vi "write_rois_to_results_file.vi"(8 "Error In":errorcluster, 9 "ROIs":T1(array[cluster]), 10 "Sample":string, 11 "File Path":path) -> (0 "Error Out":errorcluster)   [LabVIEW 2019]
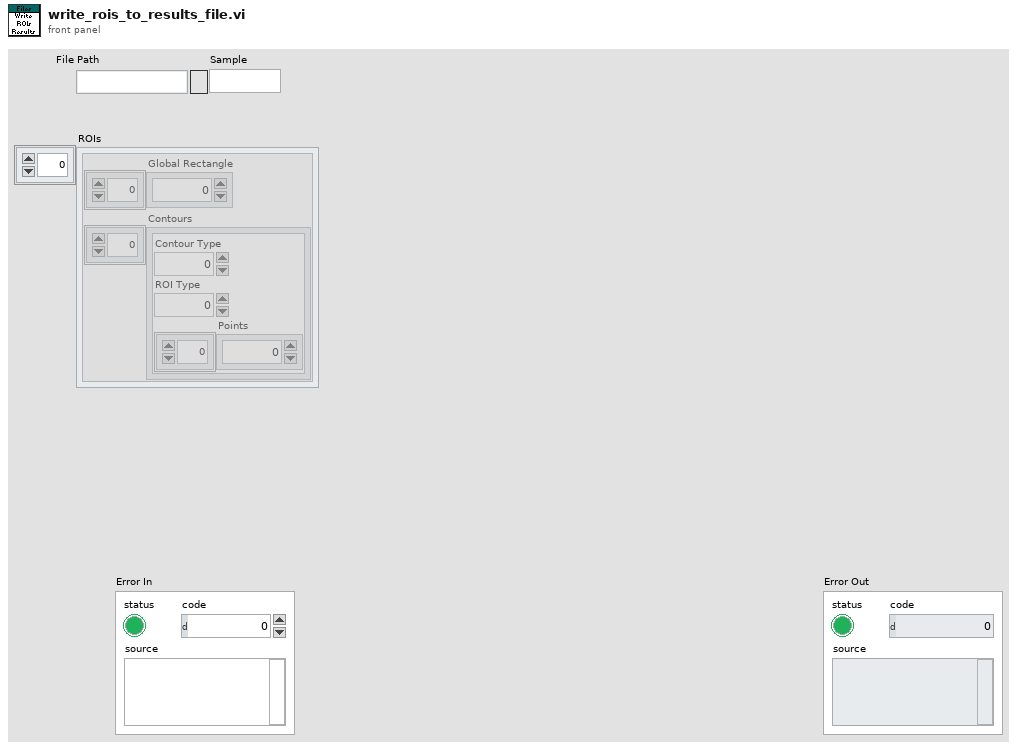
[diagram p1: front panel]
types:
  T1 = cluster{"Global Rectangle":i32[], "Contours":cluster{"Contour Type":u32, "ROI Type":u32, "Points":i32[]}[]}[]
  T2 = typedef "sample_results_cluster_typedef.ctl" = cluster{"File Path":string, "Sample":string, "Threshold":dbl, "Parameters":T3, "Writeable Parameters":T4, "Gain Results":T5[]}
  T3 = typedef "parameters_cluster_typedef.ctl" = cluster{"m1":dbl, "m2":dbl, "m3":dbl, "c":dbl, "D":dbl, "Beta":dbl, "center x":dbl, "center y":dbl}
  T4 = typedef "writeable_section_parameters_cluster_typedef.ctl" = cluster{"Section":string, "Method":i32, "Edge Mode":i32, "Grid Constant":i32, "Manual Sequence":i32, "ROI Size":i32, "Min Grain Size":dbl, "Comments":string, "File Path":string}
  T5 = typedef "grain_results_cluster_typedef.ctl" = cluster{"Grain Number":i32, "xi":dbl[], "phiin":dbl[], "Intensity":dbl[][], "Best Fit Intensity":dbl[][], "Best Fit Parameters":dbl[][], "Polarizer 1 Angle":dbl[][], "Polarizer 2 Angle":dbl[][], "Best Extinction Angle":dbl[], "Best Extinction Angle Corrected":dbl[], "Thetac":dbl, "Phic":dbl, "ROI":cluster{"Global Rectangle":i32[], "Contours":cluster{"Contour Type":u32, "ROI Type":u32, "Points":i32[]}[]}, "a":dbl, "b":dbl, "sequences available":dbl, "sequences used":dbl, "Contrast":dbl[], "Rsq":dbl}
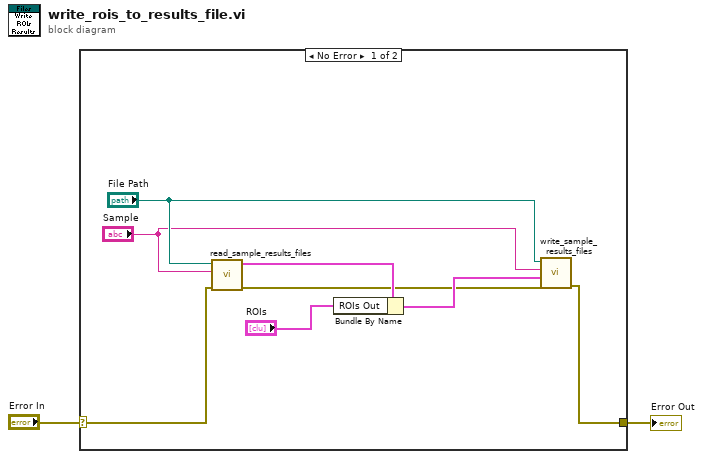
[diagram p0: block diagram]
diagram:
  n1 = case shown="No Error" "Error In" {
    selector: "Error In" -> [w6 w11]
    tunnel: [w7 w11] -> w1
    frame No Error {
      n2 = call "read_sample_results_files.vi"("Error In"=w6, "Sample"="Sample", "File Path"="File Path") -> ("Error Out"=w8:errorcluster, "Sample Results"=w10:T2)  [unwired: 7 in]
      n3 = Bundle By Name(cluster=w10, "ROIs Out"="ROIs") -> (w9:T2)
      n4 = call "write_sample_results_files.vi"("Error In"=w8, "Sample Results"=w9, "Sample"="Sample", "File Path"="File Path") -> ("Error Out"=w7:errorcluster)  [unwired: 7 in]
    }
    frame Error {
    }
  }
  "Error Out" <- w1
